vi "FetchData.vi"() -> ()   [LabVIEW 2020]
uses:
  <vilib>/addons/database/Connection.llb/Conn Execute.vi
  <vilib>/addons/database/Recordset.llb/Rec Get Recordset Properties (R).vi
  <vilib>/addons/database/Recordset.llb/Rec Fetch Recordset Data (R).vi
  <vilib>/addons/database/Recordset.llb/Rec Fetch String Data (R).vi
  <vilib>/addons/database/Recordset.llb/Rec Destroy - Connection.vi
  <vilib>/addons/database/NI_Database_API.lvlib
panel:
  out "Name":string
  out "recordset data":variant[][](array[variant])
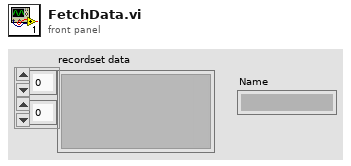
[diagram p1: front panel]
types:
  T1 = typedef "NI_Database_API.lvlib/Conn ObjectReference.ctl" = refnum<k1>
  T2 = typedef "NI_Database_API.lvlib/Rec ObjectReference.ctl" = refnum<k1>
  T3 = typedef "NI_Database_API.lvlib/Rec Properties.ctl" = cluster{"column count":i32, "record index":i32, "record count":i32, "bof?":bool, "eof?":bool, "cursor type":T4, "cache size":i32, "state":enum16{"closed", "open"}}
  T4 = typedef "NI_Database_API.lvlib/DB Tools Cursor Type.ctl" = enum16{"forward-only", "keyset", "dynamic", "static"}
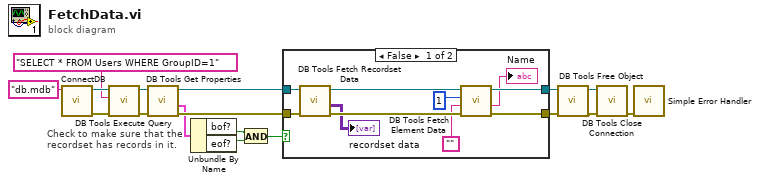
[diagram p0: block diagram]
diagram:
  # "Check to make sure that the recordset has records in it."
  n1 = call "ConnectDB.vi"("Filename"="db.mdb") -> ("error out"=w3:errorcluster, "DB Conn"=w4:T1)  [unwired: 9 in]
  n2 = call-poly <vilib>:"DB Tools Execute Query.vi"("error in (no error)"=w3, "SQL query"="SELECT * FROM Users WHERE GroupID=1", "connection reference"=w4) -> ("error out"=w16:errorcluster, "recordset reference"=w17:T2)  [unwired: 5 in]
  n3 = call-poly <vilib>:"DB Tools Get Properties.vi"("error in (no error)"=w16, "recordset reference"=w17) -> ("error out"=w14:errorcluster, "recordset properties"=w13:T3, "recordset reference out"=w15:T2)  [unwired: 3 in]
  n4 = Unbundle By Name(w13) -> ("bof?"=w11:bool, "eof?"=w10:bool)
  n5 = And(x=w11, y=w10) -> (x .and. y?=w12:bool)
  n6 = case shown="False" w12 {
    tunnel: w15 -> [w27 w29]
    tunnel: w14 -> [w26 w28]
    tunnel: [w22 w29] -> w8
    tunnel: [w23 w28] -> w9
    frame False {
      n7 = call-poly <vilib>:"DB Tools Fetch Recordset Data.vi"("error in (no error)"=w26, "recordset reference"=w27) -> ("error out"=w25:errorcluster, "recordset data"=→"recordset data":variant[][], "recordset reference out"=w24:T2)  [unwired: 3 in]
      n8 = call-poly <vilib>:"DB Tools Fetch Element Data.vi"("error in (no error)"=w25, "type"="", "column index"=1, "recordset reference"=w24) -> ("error out"=w23:errorcluster, "data"=→"Name":string, "recordset reference out"=w22:T2)  [unwired: 3 in]
    }
    frame True {
    }
  }
  n9 = call-poly <vilib>:"DB Tools Free Object.vi"("error in (no error)"=w9, "recordset reference"=w8) -> ("error out"=w6:errorcluster, "connection reference"=w7:T1)  [unwired: 8 in]
  n10 = call <vilib>:"DB Tools Close Connection.vi"("error in (no error)"=w6, "connection reference"=w7) -> ("error out"=w5:errorcluster)  [unwired: 5 in]
  n11 = call <vilib>:"Simple Error Handler.vi"("error in (no error)"=w5) -> ()  [unwired: 4 in, 5 out]
